vi "Windows Registry Manipulation.vi"() -> ()   [LabVIEW 2023]
doc: "This example demonstrates how to write, read, and delete a sample key from the Windows registry. It will not affect the registry in any other way."
uses:
  <vilib>/registry/registry.llb/Registry RtKey.ctl
  <vilib>/registry/registry.llb/Write Registry Value Simple.vi
  <vilib>/registry/registry.llb/Read Registry Value Simple.vi
panel:
  out "Sample Key Deleted?":bool
  out "Sample Key Read?":bool
  out "Sample Key Written?":bool
  # "Overview: Demonstrates the use of the Windows Registry Access VIs to write, read, and delete a sample key from the Windows registry.\nRequirements: Windows\nInstructions:\nRun the VI."
  # "See the diagram of this VI for more information on the Windows Registry Access VIs."
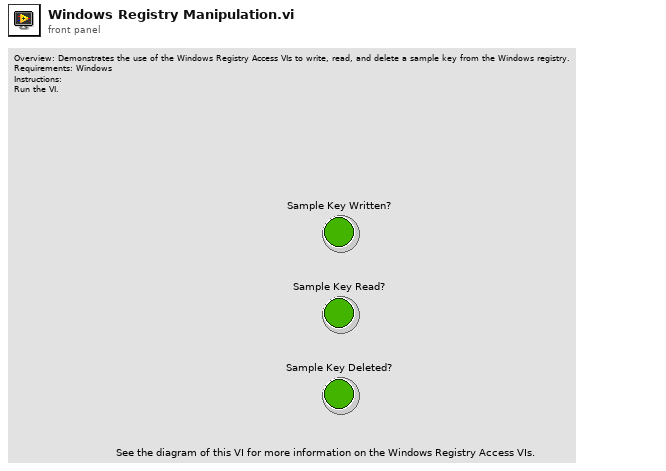
[diagram p1: front panel]
types:
  T1 = typedef "Registry RtKey.ctl" = enum32{"HKEY_CLASSES_ROOT", "HKEY_CURRENT_USER", "HKEY_LOCAL_MACHINE", "HKEY_USERS", "HKEY_PERFORMANCE_DATA", "HKEY_CURRENT_CONFIG", "HKEY_DYN_DATA"}
  T2 = typedef "Registry refnum.ctl" = refnum<k1>
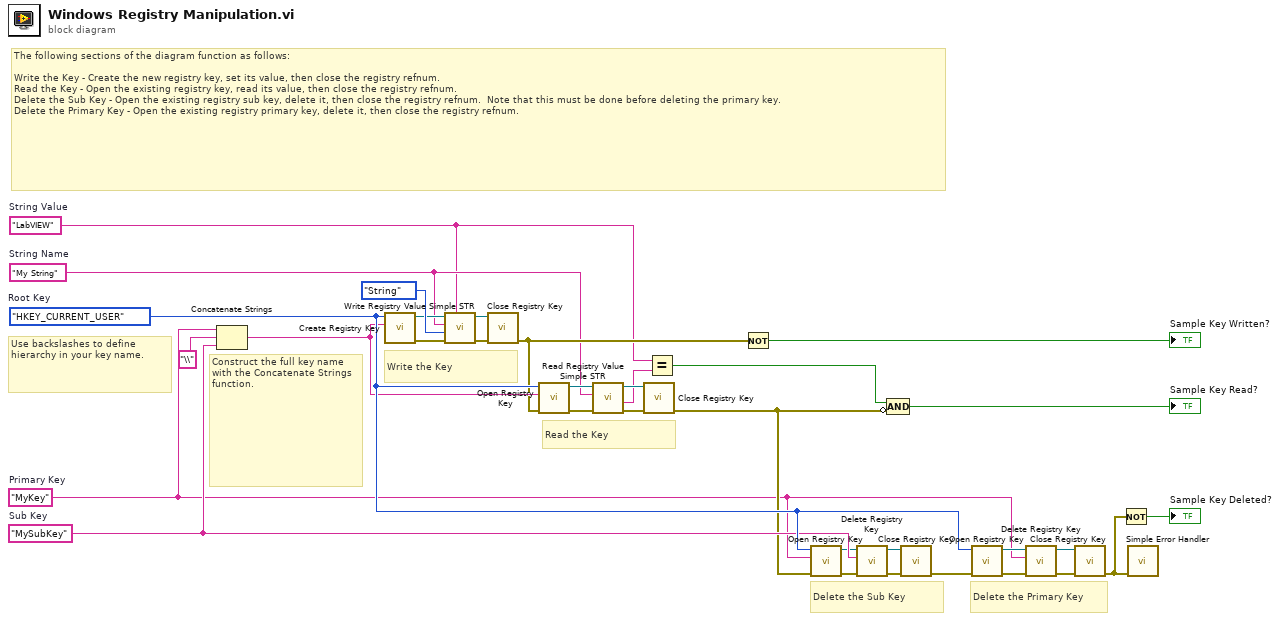
[diagram p0: block diagram]
diagram:
  w17 = "MySubKey"  # Sub Key
  w6 = "MyKey"  # Primary Key
  w7 = "LabVIEW"  # String Value
  w12 = "My String"  # String Name
  w19 = Registry_RtKey."HKEY_CURRENT_USER"  # Root Key
  # "Construct the full key name with the Concatenate Strings function."
  # "Use backslashes to define hierarchy in your key name."
  # "The following sections of the diagram function as follows:\n\nWrite the Key - Create the new registry key, set its value, then close the registry refnum.\nRead the Key - Open the existing registry key, read its value, then close the registry refnum.\nDelete the Sub Key - Open the existing registry sub key, delete it, then close the registry refnum.  Note that this must be done before deleting the primary key.\nDelete the Primary Key - Open the existing registry primary key, delete it, then close the registry refnum."
  # "Delete the Primary Key"
  # "Delete the Sub Key"
  # "Read the Key"
  # "Write the Key"
  n1 = Concatenate Strings(w6, "\\", w17) -> (w18:string)
  n2 = call <vilib>:"Create Registry Key.vi"("subkey"=w18, "root key (HKEY_LOCAL_MACHINE)"=w19) -> ("error out"=w31:errorcluster, "refnum out"=w29:T2)  [unwired: 7 in, 1 out]
  n3 = call-poly <vilib>:"Write Registry Value Simple STR.vi"("String/Binary data"=w7, "error in (no error)"=w31, "simple data type"=enum16{"String", "Binary", "DWORD"}."String", "value"=w12, "refnum"=w29) -> ("error out"=w33:errorcluster, "refnum out"=w32:T2)  [unwired: 3 in]
  n4 = call <vilib>:"Close Registry Key.vi"("error in (no error)"=w33, "refnum"=w32) -> ("error out"=w16:errorcluster)  [unwired: 5 in]
  n5 = call <vilib>:"Open Registry Key.vi"("error in (no error)"=w16, "subkey"=w18, "root key (HKEY_LOCAL_MACHINE)"=w19) -> ("error out"=w25:errorcluster, "refnum out"=w26:T2)  [unwired: 7 in]
  n6 = call-poly <vilib>:"Read Registry Value Simple STR.vi"("error in (no error)"=w25, "value"=w12, "refnum"=w26) -> ("error out"=w28:errorcluster, "String/Binary data"=w11:string, "refnum out"=w27:T2)  [unwired: 3 in, 1 out]
  n7 = call <vilib>:"Close Registry Key.vi"("error in (no error)"=w28, "refnum"=w27) -> ("error out"=w9:errorcluster)  [unwired: 5 in]
  n8 = Equal?(x=w7, y=w11) -> (x = y?=w10:bool)
  n9 = Not(x=w16) -> (.not. x?=→"Sample Key Written?":bool)
  n10 = call <vilib>:"Open Registry Key.vi"("error in (no error)"=w9, "subkey"=w6, "root key (HKEY_LOCAL_MACHINE)"=w19) -> ("error out"=w1:errorcluster, "refnum out"=w2:T2)  [unwired: 7 in]
  n11 = call <vilib>:"Delete Registry Key.vi"("error in (no error)"=w1, "subkey"=w17, "refnum"=w2) -> ("error out"=w3:errorcluster, "refnum out"=w4:T2)  [unwired: 7 in]
  n12 = Compound Arithmetic op=AND(w10, invert w9) -> (→"Sample Key Read?":bool)
  n13 = call <vilib>:"Close Registry Key.vi"("error in (no error)"=w3, "refnum"=w4) -> ("error out"=w22:errorcluster)  [unwired: 5 in]
  n14 = call <vilib>:"Open Registry Key.vi"("error in (no error)"=w22, "root key (HKEY_LOCAL_MACHINE)"=w19) -> ("error out"=w21:errorcluster, "refnum out"=w20:T2)  [unwired: 8 in]
  n15 = call <vilib>:"Delete Registry Key.vi"("error in (no error)"=w21, "subkey"=w6, "refnum"=w20) -> ("error out"=w23:errorcluster, "refnum out"=w24:T2)  [unwired: 7 in]
  n16 = call <vilib>:"Close Registry Key.vi"("error in (no error)"=w23, "refnum"=w24) -> ("error out"=w14:errorcluster)  [unwired: 5 in]
  n17 = Not(x=w14) -> (.not. x?=→"Sample Key Deleted?":bool)
  n18 = call <vilib>:"Simple Error Handler.vi"("error in (no error)"=w14) -> ()  [unwired: 4 in, 5 out]
